vi "Volt2kg.vi"(8 "error in (no error)":errorcluster, 11 "Voltage In [V]":dbl) -> (0 "error out":errorcluster, 3 "Weight Out [kg]":dbl)   [LabVIEW 2018, in "WeightMeas.lvlib"]
doc: "Converts voltage measurement into weight estimate."
uses:
  WeightMeas.lvlib
panel:
  # "Edit block diagram under the True case structure."
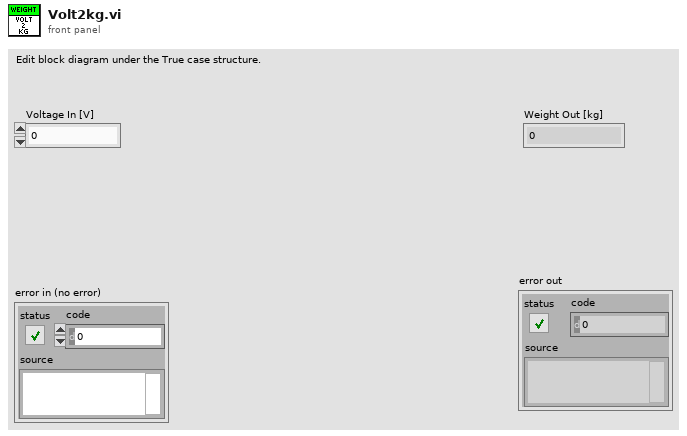
[diagram p1: front panel]
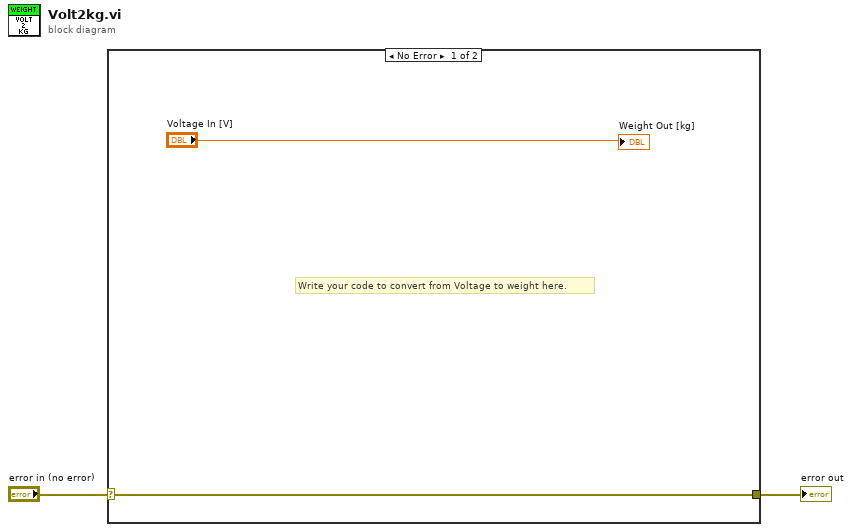
[diagram p0: block diagram]
diagram:
  n1 = case shown="No Error" "error in (no error)" {
    selector: "error in (no error)" -> [w4 w5]
    tunnel: [w4 w5] -> w1
    frame No Error {
      # "Write your code to convert from Voltage to weight here."
      "Weight Out [kg]" <- "Voltage In [V]"
    }
    frame Error {
      # "Leave empty, this case is for error handling."
    }
  }
  "error out" <- w1
